vi "limelt ctrl.vi"(8 "error in (no error)":errorcluster) -> (0 "error out":errorcluster, 3 "LimeLIGHT control":T4 {"stream" items=["standard side-by-side", "PiP Main", "PiP Secondary"]; "camMode" items=["Vision processor", "Driver Camera"]; "ledMode" items=["default to current pipeline", "force off", "force blink", "force on"]})   [LabVIEW 2023]
uses:
  ctrl defs/ctrl LIMELIGHT STREAM selector.ctl
  ctrl defs/ctrl LIMELIGHT CAMMODE selector.ctl
  ctrl defs/ctrl LIMELIGHT LEDMODE selector.ctl
  Global stack names.vi
  <vilib>/Rock Robotics/Network Tables/NT Read Boolean.vi
panel:
  out "STATE":T5(ring)
  out "LOOKING\nfor NOTE?":bool
  out "NOTE\nLOADED?":bool
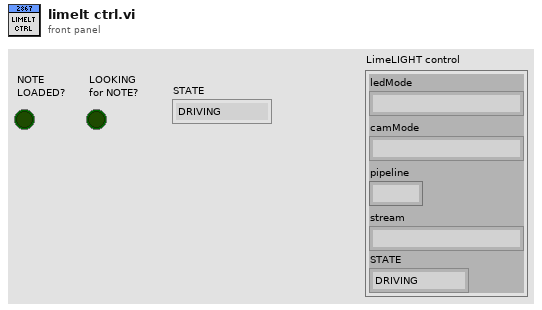
[diagram p1: front panel]
types:
  T1 = typedef "ctrl LIMELIGHT STREAM selector.ctl" = u16
  T2 = typedef "ctrl LIMELIGHT CAMMODE selector.ctl" = u16
  T3 = typedef "ctrl LIMELIGHT LEDMODE selector.ctl" = u16
  T4 = cluster{"stream":T1, "pipeline":u16, "camMode":T2, "ledMode":T3, "STATE":enum16{"DRIVING", "LOOKING for NOTE", "HAVE NOTE"}}
  T5 = enum16{"DRIVING", "LOOKING for NOTE", "HAVE NOTE"}
  T6 = typedef "ctrl stack - INTAKE SHOOTER.ctl" = cluster{"INTAKE STATE":string, "RUN INTAKE?":string, "RUN REVERSE?":string, "NOTE LOADED?":string, "SHOOTER STATE":string, "SHOOTER FIRE?":string, "SHOOT AMP?":string, "EXTEND FLAP?":string, "LOOKING for NOTE":string, "OVERIDE NOTE CHECK":string}
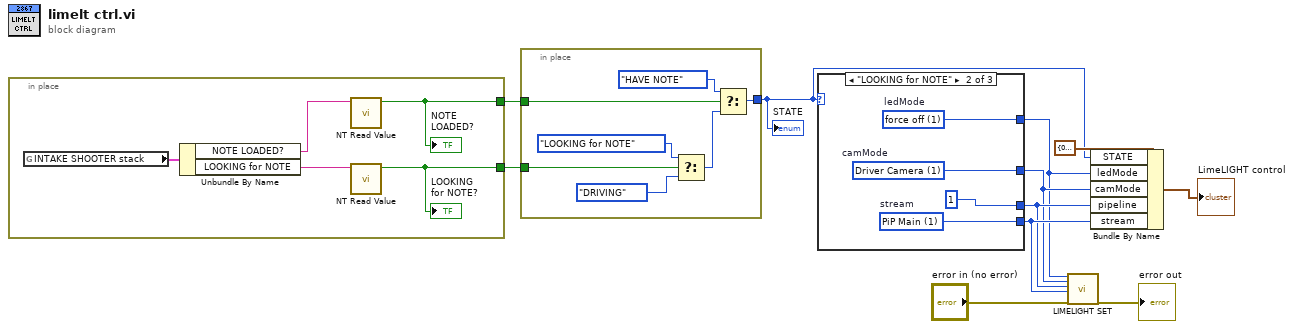
[diagram p0: block diagram]
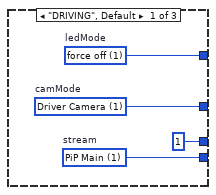
[diagram p2: hidden frame]
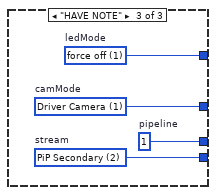
[diagram p3: hidden frame]
diagram:
  n1 = in-place {
    in-place-border: [w13] -> w11
    in-place-border: [w12] -> w10
    n2 = global read "Global stack names.vi" "INTAKE SHOOTER stack"() -> (w16:T6)
    n3 = Unbundle By Name(w16) -> ("NOTE LOADED?"=w15:string, "LOOKING for NOTE"=w14:string)
    n4 = call-poly <vilib>:"NT Read Value.vi"("name"=w15) -> ("value"=w12:bool)  [unwired: 8 in, 2 out]
    "NOTE\nLOADED?" <- w12
    n5 = call-poly <vilib>:"NT Read Value.vi"("name"=w14) -> ("value"=w13:bool)  [unwired: 8 in, 2 out]
    "LOOKING\nfor NOTE?" <- w13
  }
  n6 = in-place {
    in-place-border: w11 -> [w21]
    in-place-border: w10 -> [w20]
    in-place-border: [w17] -> w1
    n7 = Select(t=T5."LOOKING for NOTE" ("STATE"), s=w21, f=T5."DRIVING" ("STATE")) -> (s? t:f=w18:T5)
    n8 = Select(t=T5."HAVE NOTE" ("STATE"), s=w20, f=w18) -> (s? t:f=w17:T5)
  }
  "STATE" <- w1
  n9 = case shown="\"LOOKING for NOTE\"" w1 {
    tunnel: [w25 w31 w35] -> w2
    tunnel: [w26 w30 w34] -> w3
    tunnel: [u16 1 ("pipeline") u16 1 ("pipeline") w33] -> w4
    tunnel: [w27 w29 w32] -> w5
    frame "DRIVING", Default {
      w25 = T3 1 items=["default to current pipeline", "force off", "force blink", "force on"]  # ledMode
      w26 = T2 1 items=["Vision processor", "Driver Camera"]  # camMode
      w27 = T1 1 items=["standard side-by-side", "PiP Main", "PiP Secondary"]  # stream
    }
    frame "LOOKING for NOTE" {
      w29 = T1 1 items=["standard side-by-side", "PiP Main", "PiP Secondary"]  # stream
      w30 = T2 1 items=["Vision processor", "Driver Camera"]  # camMode
      w31 = T3 1 items=["default to current pipeline", "force off", "force blink", "force on"]  # ledMode
    }
    frame "HAVE NOTE" {
      w32 = T1 2 items=["standard side-by-side", "PiP Main", "PiP Secondary"]  # stream
      w33 = u16 1  # pipeline
      w34 = T2 1 items=["Vision processor", "Driver Camera"]  # camMode
      w35 = T3 1 items=["default to current pipeline", "force off", "force blink", "force on"]  # ledMode
    }
  }
  n10 = call "LIMELIGHT SET.vi"("ledMode"=w2, "camMode"=w3, "pipeline"=w4, "stream"=w5, "error in (no error)"="error in (no error)") -> ("error out"=→"error out":errorcluster)  [unwired: 14 in]
  n11 = Bundle By Name(cluster=T4 {"stream"=0, "pipeline"=0, "camMode"=0, "ledMode"=0, "STATE"=enum."DRIVING"} ("LimeLIGHT control"), "STATE"=w1, "ledMode"=w2, "camMode"=w3, "pipeline"=w4, "stream"=w5) -> (→"LimeLIGHT control":T4)
